vi "Eval Func at Sampling Pnts (VI).vi"(6 "data":variant, 7 "f(x)":refnum<vi>, 8 "error in (no error)":errorcluster, 10 "lower limit":dbl, 11 "upper limit":dbl) -> (0 "error out":errorcluster, 2 "Sampling points (7-order)":dbl[](array[numeric]), 3 "Function Evaluations (7 and 4 pts)":dbl[](array[numeric]))   [LabVIEW 2017, in "NI_AALPro.lvlib"]
uses:
  NI_AALPro.lvlib
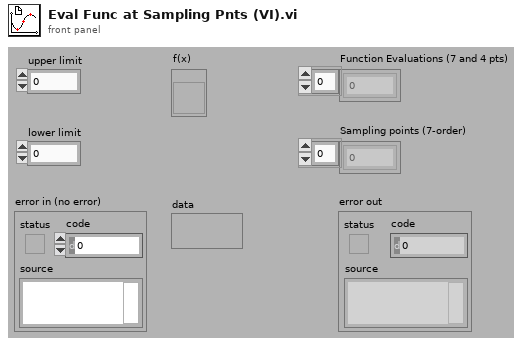
[diagram p1: front panel]
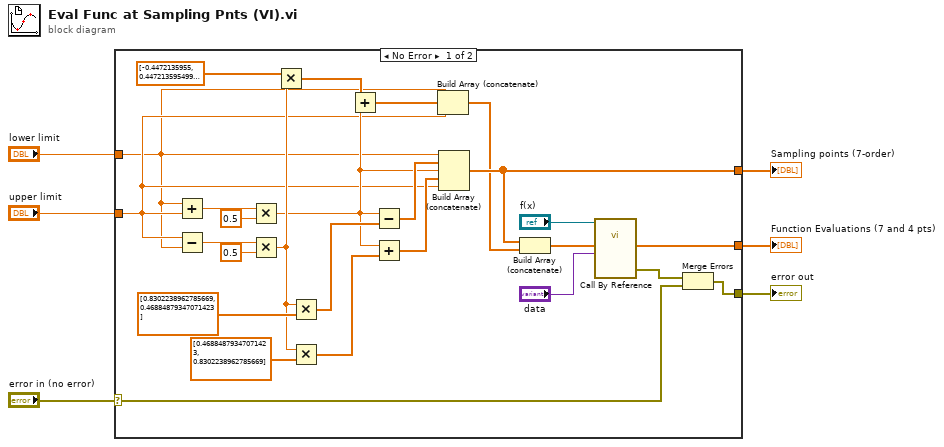
[diagram p0: block diagram]
diagram:
  n1 = case shown="No Error" "error in (no error)" {
    selector: "error in (no error)" -> [w8 w33]
    tunnel: [w17 _] -> w6
    tunnel: [w11 _] -> w5
    tunnel: [w10 w33] -> w4
    tunnel: "lower limit" -> [w14 _]
    tunnel: "upper limit" -> [w18 _]
    frame No Error {
      n2 = Add(x=w14, y=w18) -> (x+y=w28:dbl)
      n3 = Subtract(x=w18, y=w14) -> (x-y=w26:dbl)
      n4 = Multiply(x=w28, y=0.5) -> (x*y=w20:dbl)
      n5 = Multiply(x=w26, y=0.5) -> (x*y=w22:dbl)
      n6 = Multiply(x=dbl[] [-0.4472135955, 0.4472135954999579] ("appended array"), y=w22) -> (x*y=w21:dbl[])
      n7 = Multiply(x=w22, y=dbl[] [0.8302238962785669, 0.46884879347071423] ("appended array")) -> (x*y=w32:dbl[])
      n8 = Multiply(x=w22, y=dbl[] [0.46884879347071423, 0.8302238962785669] ("appended array")) -> (x*y=w31:dbl[])
      n9 = Add(x=w21, y=w20) -> (x+y=w19:dbl[])
      n10 = Subtract(x=w20, y=w32) -> (x-y=w30:dbl[])
      n11 = Add(x=w20, y=w31) -> (x+y=w29:dbl[])
      n12 = Build Array (concatenate)(w14, w19, w18) -> (w16:dbl[])
      n13 = Build Array (concatenate)(w14, w30, w20, w29, w18) -> (w17:dbl[])
      n14 = Build Array (concatenate)(w17, w16) -> (w12:dbl[])
      n15 = call-by-ref "?"(reference="f(x)", "Variant"="data", "Array"=w12) -> ("error out"=w9:errorcluster, "Array 2"=w11:dbl[])  [unwired: 9 in, 2 out]
      n16 = Merge Errors(w9, w8) -> (w10:errorcluster)
    }
    frame Error {
    }
  }
  "Sampling points (7-order)" <- w6
  "Function Evaluations (7 and 4 pts)" <- w5
  "error out" <- w4
